vi "CCT calculator.vi"(10 "n":dbl) -> (2 "CCT":dbl)   [LabVIEW 2014, in "AMS TS3472 Light Sensor.lvlib" / "AMS TCS3472.lvclass"]
uses:
  AMS TCS3472.lvclass
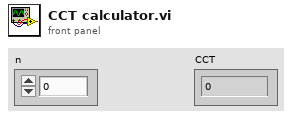
[diagram p1: front panel]
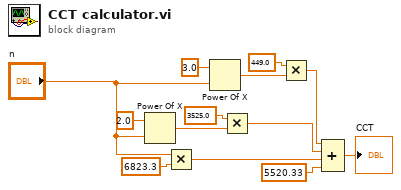
[diagram p0: block diagram]
diagram:
  n1 = Power Of X(1:"n", 2:2.0 ("y")) -> (0:w6:dbl)
  n2 = Multiply(x="n", y=6823.3) -> (x*y=w1:dbl)
  n3 = Power Of X(1:"n", 2:3.0 ("y")) -> (0:w9:dbl)
  n4 = Multiply(x=3525.0, y=w6) -> (x*y=w4:dbl)
  n5 = Multiply(x=449.0, y=w9) -> (x*y=w7:dbl)
  n6 = Compound Arithmetic op=ADD(w7, w4, w1, 5520.33 ("value")) -> (→"CCT":dbl)
